vi "TestManyPublications.vi"(8 "error in (no error)":errorcluster, 11 "TestPublishRate In":refnum<class "TestManyPublications.lvclass">) -> (0 "error out":errorcluster, 3 "TestPublishRate Out":refnum<class "TestManyPublications.lvclass">)   [LabVIEW 2015, in "TestManyPublications.lvclass"]
uses:
  TestManyPublications.lvclass
  Framework/IViewModel/IViewModel/IViewModel.lvclass
  Framework/IViewable/IViewable/IViewable.lvclass
  Doubles/TestModelManyTopics/TestModelManyTopics.lvclass
  Framework/Mediator/Mediator/Mediator.lvclass
  Framework/SubscriptionPolicy/ValueChangeSubscription/ValueChangeSubscription.lvclass/ValueChangeSubscription.ctl
  Framework/IViewModel/IViewModel/IViewModel.lvclass/IViewModel.ctl
  Framework/IViewManager/IViewManager Messages/Launch Nested Views Msg/Launch Nested Views Msg.lvclass/Launch Nested Views Msg.ctl
  Framework/IViewManager/IViewManager/IViewManager.lvclass/IViewManager.ctl
  Framework/IObserver/IObserver Messages/Subscribe Msg/Subscribe Msg.lvclass/Subscribe Msg.ctl
  <vilib>/ActorFramework/Message Enqueuer/Message Enqueuer.lvclass/Message Enqueuer.ctl
  <vilib>/ActorFramework/Stop Msg/Stop Msg.lvclass/Stop Msg.ctl
  Framework/IViewManager/IViewManager Messages/Launch Nested Views Msg/Build Launch Nested Views Msg.vi
  Framework/IViewManager/IViewManager/Write Startup Launch Nested Views Msg.vi
  <vilib>/ActorFramework/Message Enqueuer/Enqueue.vi
  <vilib>/ActorFramework/Message Enqueuer/Enqueue Critical.vi
  <vilib>/ActorFramework/Message Priority Queue/Priority Enqueue.vi
  Framework/IViewManager/IViewManager Messages/Launch Nested Views Msg/Launch Nested Views Msg.lvclass
  Framework/SubscriptionPolicy/ValueChangeSubscription/ValueChangeSubscription.lvclass
  Framework/IObserver/IObserver Messages/Subscribe Msg/Subscribe Msg.lvclass
  <vilib>/ActorFramework/Stop Msg/Stop Msg.lvclass
  Framework/Transport/QueueTransport/QueueTransport.lvclass
  <vilib>/ActorFramework/Actor/Actor.lvclass
  Framework/IMediator/SubscriptionRequest/SubscriptionRequest.lvclass
  Framework/IMediator/ISubscriptionPolicy/ISubscriptionPolicy.lvclass
panel:
  out "Final Sample Transmission Time":dbl
  out "Topic 599 Transmission Time":dbl[](graph)
  out "Iteration":i32
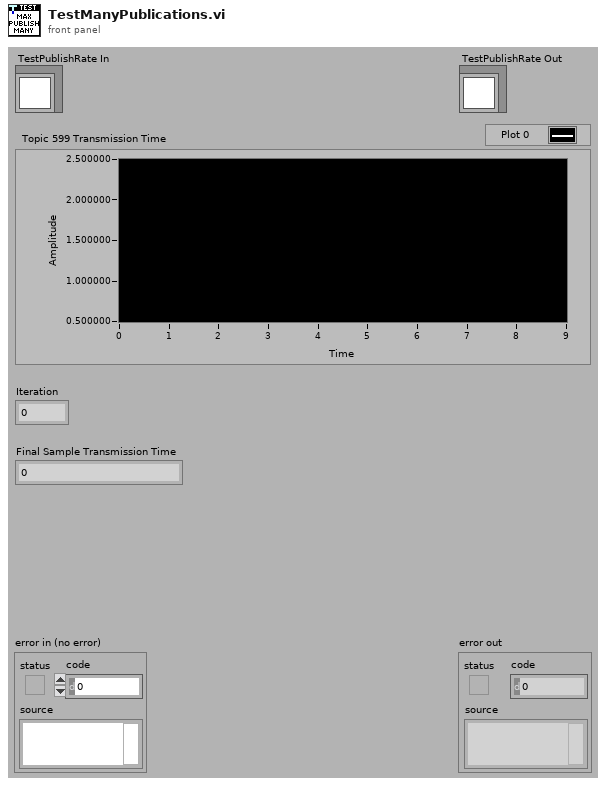
[diagram p1: front panel]
types:
  T1 = typedef "IMediator.lvlib/ISubscriptionPolicy.lvclass/ISubscriptionPolicy Reference.ctl" = refnum<data-value>
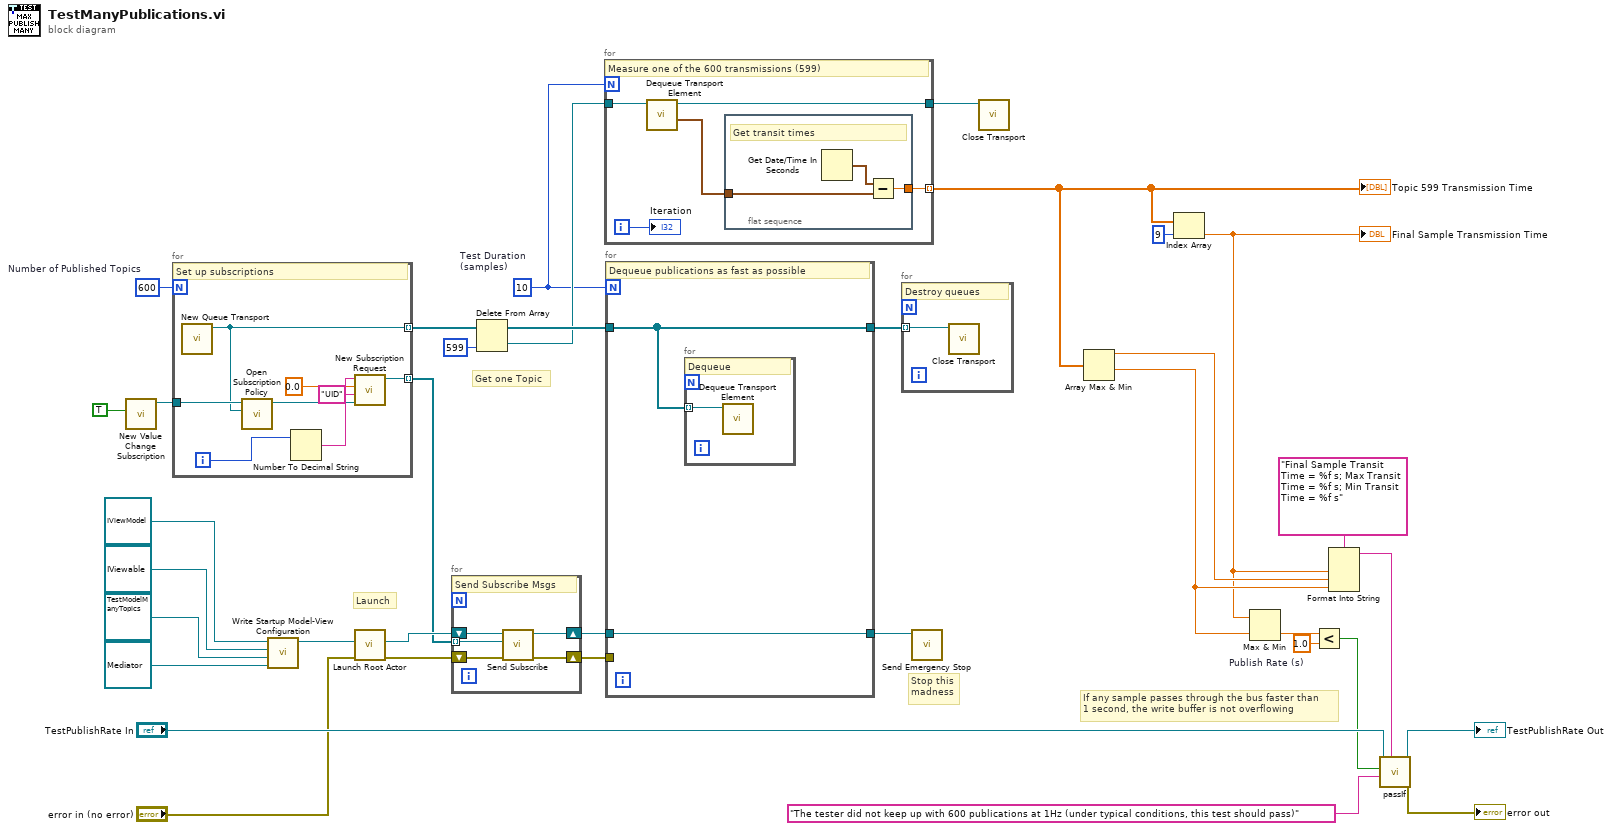
[diagram p0: block diagram]
diagram:
  w2 = 1.0  # Publish Rate (s)
  w18 = 600  # Number of Published Topics
  w10 = 10  # Test Duration (samples)
  # "If any sample passes through the bus faster than\n1 second, the write buffer is not overflowing"
  # "Get one Topic"
  # "Stop this\nmadness"
  # "Launch"
  n1 = call "New Value Change Subscription.vi"("Ignore Past Updates? (F)"=TRUE) -> ("ValueChangeSubscription Out"=w16:refnum<class "ValueChangeSubscription.lvclass">)  [unwired: 10 in]
  n2 = for {
    N: w18 -> [_]
    tunnel: [w42] -> w26 mode=indexing
    tunnel: w16 -> [w40]
    tunnel: [w37] -> w15 mode=indexing
    i -> [w39]
    # "Set up subscriptions"
    n3 = call "New Queue Transport.vi"() -> ("QueueTransport Out"=w37:refnum<class "QueueTransport.lvclass">)  [unwired: 10 in, 1 out]
    n4 = call "Open Subscription Policy.vi"("Transport"=w37, "SubscriptionPolicy"=w40) -> ("Subscription Policy"=w44:T1)  [unwired: 8 in, 1 out]
    n5 = Number To Decimal String(number=w39) -> (decimal integer string=w38:string)  [unwired: 1 in]
    n6 = call "New Subscription Request.vi"("Subscription Policy"=w44, "Subscriber ID"="UID" ("Unique Subscriber ID"), "Type"=0.0, "Datum Name"=w38) -> ("SubscriptionRequest"=w42:refnum<class "SubscriptionRequest.lvclass">)  [unwired: 7 in]
  }
  n7 = call "Write Startup Model-View Configuration.vi"("Mediator Type"=refnum<class "Mediator.lvclass"> refnum ("Mediator"), "Model Type"=refnum<class "TestModelManyTopics.lvclass"> refnum ("Model"), "Startup View Configuration"=refnum<class "IViewable.lvclass"> refnum, "IViewModel In"=refnum<class "IViewModel.lvclass"> refnum) -> ("IViewModel Out"=w28:refnum<class "IViewModel.lvclass">)  [unwired: 7 in]
  n8 = call <vilib>:"Launch Root Actor.vi"("error in (no error)"="error in (no error)", "Actor"=w28) -> ("error out"=w24:errorcluster, "Actor's Enqueuer"=w27:refnum<class "Message Enqueuer.lvclass">)  [unwired: 8 in]
  n9 = for {
    tunnel: w26 -> [w48] mode=indexing
    shift-right: [w47] -> w25
    shift-left: w27 -> [w49]
    shift-right: [w45] -> w23
    shift-left: w24 -> [w46]
    # "Send Subscribe Msgs"
    n10 = call "Send Subscribe.vi"("error in (no error)"=w46, "SubscriptionRequest"=w48, "Message Enqueuer"=w49) -> ("error out"=w45:errorcluster, "Message Enqueuer out"=w47:refnum<class "Message Enqueuer.lvclass">)  [unwired: 7 in]
  }
  n11 = Delete From Array(array=w15, index=599) -> (deleted portion=w12:refnum<class "QueueTransport.lvclass">, array with subset deleted=w13:refnum<class "QueueTransport.lvclass">[])  [unwired: 1 in]
  n12 = for {
    N: w10 -> [_]
    tunnel: w12 -> [w54]
    tunnel: [w53] -> w11
    tunnel: [w52] -> w7 mode=indexing
    i -> [w51]
    # "Measure one of the 600 transmissions (599)"
    n13 = call "Dequeue Transport Element.vi"("QueueTransport in"=w54) -> ("Publication Time"=w50:timestamp, "QueueTransport out"=w53:refnum<class "QueueTransport.lvclass">)  [unwired: 7 in, 2 out]
    n14 = flat-sequence {
      tunnel: [w56] -> w52
      tunnel: w50 -> [w55]
      frame #0 {
        # "Get transit times"
        n15 = Get Date/Time In Seconds() -> (seconds since 1Jan1904=w57:timestamp)
        n16 = Subtract(x=w57, y=w55) -> (x-y=w56:dbl)
      }
    }
    "Iteration" <- w51
  }
  "Topic 599 Transmission Time" <- w7
  n17 = for {
    N: w10 -> [_]
    tunnel: w25 -> [w59]
    tunnel: w23 -> [_]
    tunnel: [w59] -> w22
    tunnel: [w58] -> w21
    tunnel: w13 -> [w58]
    # "Dequeue publications as fast as possible"
    n18 = for {
      tunnel: w58 -> [w60] mode=indexing
      # "Dequeue"
      n19 = call "Dequeue Transport Element.vi"("QueueTransport in"=w60) -> ()  [unwired: 7 in, 4 out]
    }
  }
  n20 = for {
    tunnel: w21 -> [w61] mode=indexing
    # "Destroy queues"
    n21 = call-dynamic "Close Transport.vi"("QueueTransport in"=w61) -> ()  [unwired: 10 in, 1 out]
  }
  n22 = call <vilib>:"Send Emergency Stop.vi"("Message Enqueuer"=w22) -> ()  [unwired: 10 in, 1 out]
  n23 = call-dynamic "Close Transport.vi"("QueueTransport in"=w11) -> ()  [unwired: 10 in, 1 out]
  n24 = Array Max & Min(array=w7) -> (max value=w6:dbl, min value=w5:dbl)  [unwired: 2 out]
  n25 = Index Array(array=w7, index=9) -> (element=w4:dbl)
  "Final Sample Transmission Time" <- w4
  n26 = Max & Min(x=w4, y=w5) -> (min(x,y)=w3:dbl)  [unwired: 1 out]
  n27 = Less?(x=w3, y=w2) -> (x < y?=w1:bool)
  n28 = Format Into String(format string="Final Sample Transit Time = %f s; Max Transit Time = %f s; Min Transit Time = %f s", w4, w6, w5) -> (resulting string=w20:string)  [unwired: 2 in, 1 out]
  n29 = call-dynamic "passIf.vi"("custom report message (\"\")"=w20, "message (\"\")"="The tester did not keep up with 600 publications at 1Hz (under typical conditions, this test should pass)" ("message (\"\")"), "pass"=w1, "TestCase in"="TestPublishRate In") -> ("error out"=→"error out":errorcluster, "TestCase out"=→"TestPublishRate Out":refnum<class "TestManyPublications.lvclass">)  [unwired: 6 in]
